vi "SupplementalDataFileNode_Entry_V2.vi"(8 "error in (no error)":errorcluster, 10 "actual count":i32, 11 "Byte Stream File in":refnum<file>) -> (0 "error out":errorcluster, 3 "Byte Stream File out":refnum<file>)   [LabVIEW 2019]
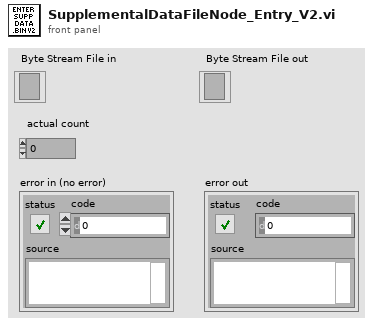
[diagram p1: front panel]
types:
  T1 = enum16{"big-endian, network order", "native, host order", "little-endian"}
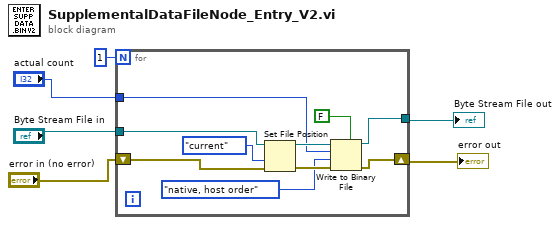
[diagram p0: block diagram]
diagram:
  n1 = for {
    N: 1 -> [_]
    shift-right: [w12] -> w5
    shift-left: "error in (no error)" -> [w13]
    tunnel: "Byte Stream File in" -> [w9]
    tunnel: [w8] -> w1
    tunnel: "actual count" -> [w7]
    n2 = Set File Position(refnum=w9, from (0:start)=enum16{"start", "end", "current"}."current", error in=w13) -> (refnum out=w15:refnum<file>, error out=w14:errorcluster)  [unwired: 1 in]
    n3 = Write to Binary File(file (use dialog)=w15, data=w7, error in=w14, 5:FALSE ("prepend array or string size? (T)"), 9:T1."native, host order" ("byte order (0:big-endian, network order)")) -> (refnum out=w8:refnum<file>, error out=w12:errorcluster)  [unwired: 1 in, 1 out]
  }
  "error out" <- w5
  "Byte Stream File out" <- w1
